vi "DB Test.vi"() -> ()   [LabVIEW 2015, in "FileHandler.lvlib"]
uses:
  FileHandler.lvlib
  <vilib>/drjdpowell/SQLite Library/SQL Statement/SQL Statement.lvclass/SQL Statement.ctl
  <vilib>/drjdpowell/SQLite Library/SQL Connection/Open (path).vi
  <vilib>/drjdpowell/SQLite Library/SQL Statement/Bind Timestamp (Text).vi
  <vilib>/drjdpowell/SQLite Library/SQL Statement/Bind Path.vi
  <vilib>/drjdpowell/SQLite Library/SQL Connection/Open (string).vi
  <vilib>/drjdpowell/SQLite Library/SQL Statement/Step.vi
  <vilib>/drjdpowell/SQLite Library/SQL Statement/Bind Text.vi
  <vilib>/drjdpowell/SQLite Library/SQL Statement/Bind Null.vi
  <vilib>/AdvancedString/Path To Command Line String.vi
  <vilib>/drjdpowell/SQLite Library/SQL Connection/Execute SQL (No results).vi
  <vilib>/drjdpowell/SQLite Library/SQL Statement/Error Message.vi
  <vilib>/drjdpowell/SQLite Library/SQL Connection/Connection.lvclass
  <vilib>/drjdpowell/SQLite Library/SQLite.lvlib
  <vilib>/drjdpowell/SQLite Library/SQL Statement/SQL Statement.lvclass
panel:
  in  "Path":path
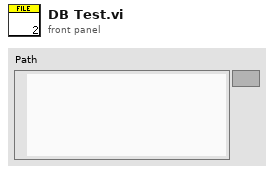
[diagram p1: front panel]
types:
  T1 = enum16{"New or existing", "Existing", "Read only"}
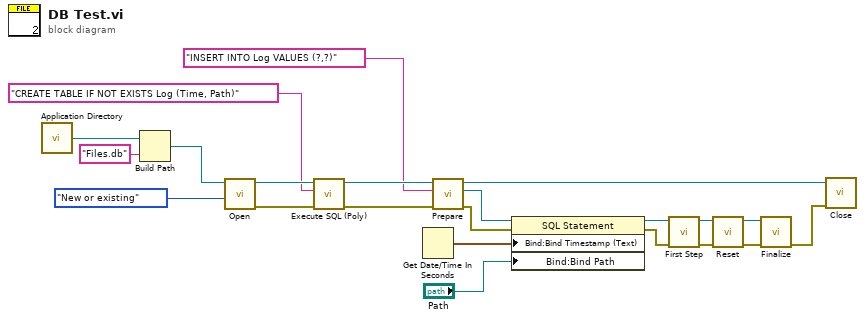
[diagram p0: block diagram]
diagram:
  n1 = call <vilib>:"Application Directory.vi"() -> ("Application Directory"=w21:path)
  n2 = Build Path(base path=w21, name or relative path="Files.db") -> (appended path=w19:path)
  n3 = call-poly <vilib>:"Open.vi"("File Option"=T1."New or existing", "db file"=w19) -> ("error out"=w17:errorcluster, "SQLite Connection out"=w18:refnum<class "Connection.lvclass">)  [unwired: 8 in]
  n4 = call-poly <vilib>:"Execute SQL (Poly).vi"("error in (no error)"=w17, "SQL"="CREATE TABLE IF NOT EXISTS Log (Time, Path)", "SQLite Connection in"=w18) -> ("error out"=w14:errorcluster, "SQLite Connection out"=w15:refnum<class "Connection.lvclass">)  [unwired: 7 in]
  n5 = Get Date/Time In Seconds() -> (seconds since 1Jan1904=w10:timestamp)
  n6 = call <vilib>:"Prepare.vi"("error in (no error)"=w14, "SQL"="INSERT INTO Log VALUES (?,?)", "SQLite Connection in"=w15) -> ("error out"=w12:errorcluster, "SQL Statement out"=w11:refnum<class "SQL Statement.lvclass">, "SQLite Connection out"=w2:refnum<class "Connection.lvclass">)  [unwired: 4 in, 2 out]
  n7 = property class="SQL Statement"(reference=w11, error in=w12, "Bind:Bind Timestamp (Text)"=w10, "Bind:Bind Path"="Path") -> (reference out=w7:refnum<class "SQL Statement.lvclass">, error out=w6:errorcluster)
  n8 = call <vilib>:"First Step.vi"("error in (no error)"=w6, "SQL Statement in"=w7) -> ("error out"=w5:errorcluster, "SQL Statement out"=w8:refnum<class "SQL Statement.lvclass">)  [unwired: 7 in, 1 out]
  n9 = call <vilib>:"Reset.vi"("error in (no error)"=w5, "SQL Statement in"=w8) -> ("error out"=w3:errorcluster, "SQL Statement out"=w4:refnum<class "SQL Statement.lvclass">)  [unwired: 8 in]
  n10 = call <vilib>:"Finalize.vi"("error in (no error)"=w3, "SQL Statement in"=w4) -> ("error out"=w1:errorcluster)  [unwired: 9 in]
  n11 = call-dynamic "Close.vi"("error in (no error)"=w1, "SQLite Connection in"=w2) -> ()  [unwired: 9 in, 1 out]
